vi "Local Transition Outward.vi"(8 "error in (no error)":errorcluster, 11 "State Machine in":refnum<class "State Machine.lvclass">) -> (0 "error out":errorcluster, 3 "State Machine out":refnum<class "State Machine.lvclass">)   [LabVIEW 2024, in "State Pattern Actor.lvlib" / "State Machine.lvlib" / "State Machine.lvclass"]
uses:
  State Machine.lvclass
  State Machine.lvclass/State Machine.ctl
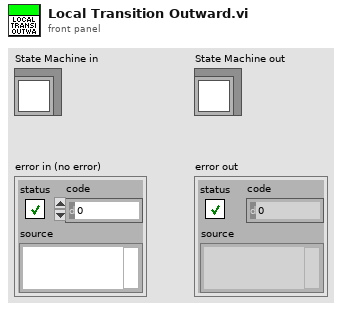
[diagram p1: front panel]
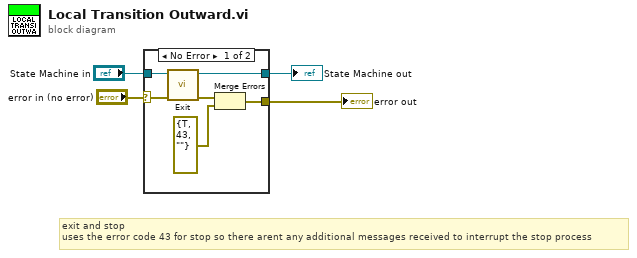
[diagram p0: block diagram]
diagram:
  # "exit and stop\nuses the error code 43 for stop so there arent any additional messages received to interrupt the stop process"
  n1 = case shown="No Error" "error in (no error)" {
    selector: "error in (no error)" -> [w8 w12]
    tunnel: [w5 w12] -> w3
    tunnel: [w9 w11] -> w1
    tunnel: "State Machine in" -> [w10 w11]
    frame No Error {
      n2 = call-dynamic "Exit.vi"("error in (no error)"=w8, "State Machine in"=w10) -> ("error out"=w7:errorcluster, "State Machine out"=w9:refnum<class "State Machine.lvclass">)  [unwired: 8 in]
      n3 = Merge Errors(w7, errorcluster {"status"=TRUE, "code"=43, "source"=""} ("error constant")) -> (w5:errorcluster)
    }
    frame Error {
    }
  }
  "error out" <- w3
  "State Machine out" <- w1
